vi "UI - Initiate Connection.vi"(8 "error in (no error)":errorcluster, 10 "Controller Address":string, 11 "Message Queue":refnum<queue>) -> (0 "error out":errorcluster, 1 "Connected?":bool, 3 "dup Message Queue":refnum<queue>)   [LabVIEW 2013]
uses:
  Message Queue/Message Cluster.ctl
  controls/Variable References.ctl
  Globals/Global - Configuration Options.vi
  Globals/Global - UI Stream and Variable Connections.vi
  Message Queue/Message Queue.lvlib
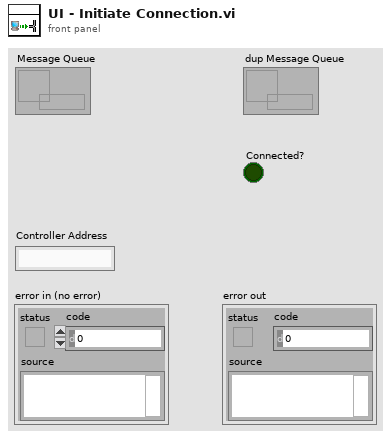
[diagram p1: front panel]
types:
  T1 = typedef "Message Queue.lvlib/Message Cluster.ctl" = cluster{"Message":string, "Message Data":variant}
  T2 = typedef "Variable References.ctl" = cluster{"CPU Usage":refnum<k21>, "Contiguous Memory":refnum<k21>, "Buffer Backlog":refnum<k21>, "Drive Space":refnum<k21>, "Number of Data Files":refnum<k21>, "System Time":refnum<k21>}
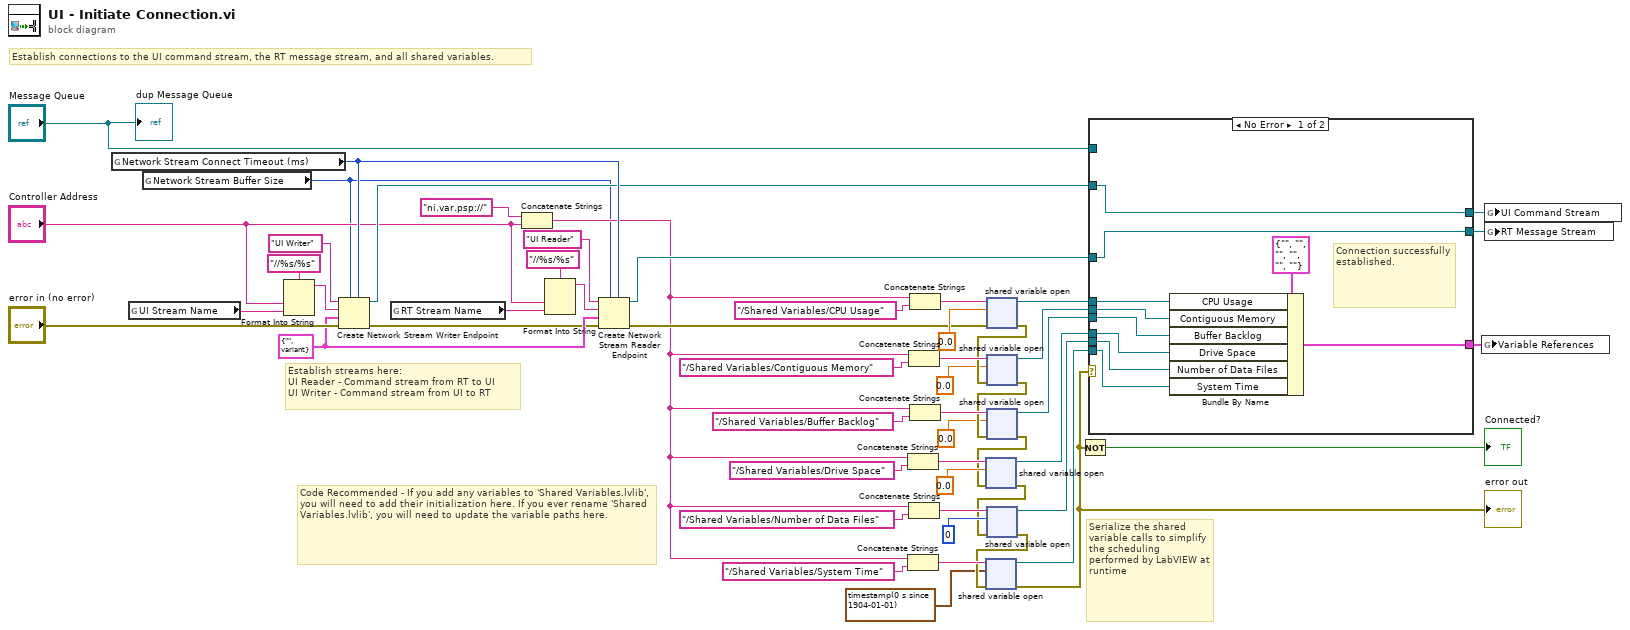
[diagram p0: block diagram]
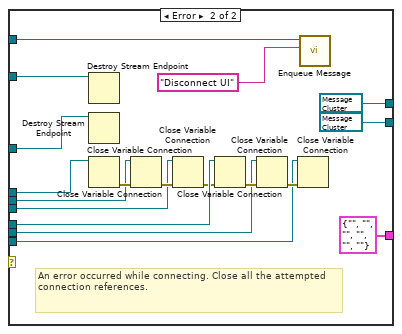
[diagram p2: hidden frame]
diagram:
  w44 = T1 {"Message"="", "Message Data"=variant} ("Message Cluster")
  # "Establish connections to the UI command stream, the RT message stream, and all shared variables."
  # "Code Recommended - If you add any variables to 'Shared Variables.lvlib', you will need to add their initialization here. If you ever rename 'Shared Variables.lvlib', you will need to update the variable paths here."
  # "Establish streams here:\nUI Reader - Command stream from RT to UI\nUI Writer - Command stream from UI to RT"
  # "Serialize the shared variable calls to simplify the scheduling performed by LabVIEW at runtime"
  n1 = global read "Global - Configuration Options.vi" "Network Stream Connect Timeout (ms)"() -> (w42:i32)
  n2 = global read "Global - Configuration Options.vi" "UI Stream Name"() -> (w49:string)
  n3 = global read "Global - Configuration Options.vi" "Network Stream Buffer Size"() -> (w3:i32)
  n4 = Format Into String(format string="//%s/%s", "Controller Address", w49) -> (resulting string=w48:string)  [unwired: 2 in, 1 out]
  n5 = Create Network Stream Writer Endpoint(5:w42, 7:w3, 8:"error in (no error)", 9:w44, 10:w48, 11:"UI Writer" ("reader name")) -> (0:w43:errorcluster, 3:w26:refnum<k21>)  [unwired: 1 in]
  n6 = global read "Global - Configuration Options.vi" "RT Stream Name"() -> (w52:string)
  n7 = Concatenate Strings("ni.var.psp://", "Controller Address") -> (w7:string)
  n8 = Format Into String(format string="//%s/%s", "Controller Address", w52) -> (resulting string=w51:string)  [unwired: 2 in, 1 out]
  n9 = Create Network Stream Reader Endpoint(5:w42, 7:w3, 8:w43, 9:w44, 10:w51, 11:"UI Reader" ("writer name")) -> (0:w39:errorcluster, 3:w27:refnum<k21>)  [unwired: 1 in]
  n10 = Concatenate Strings(w7, "/Shared Variables/Drive Space") -> (w19:string)
  n11 = Concatenate Strings(w7, "/Shared Variables/System Time") -> (w11:string)
  n12 = Concatenate Strings(w7, "/Shared Variables/Contiguous Memory") -> (w35:string)
  n13 = Concatenate Strings(w7, "/Shared Variables/Number of Data Files") -> (w14:string)
  n14 = Concatenate Strings(w7, "/Shared Variables/CPU Usage") -> (w38:string)
  n15 = Concatenate Strings(w7, "/Shared Variables/Buffer Backlog") -> (w34:string)
  n16 = shared-variable-open(w38, w39, 0.0) -> (w30:refnum<k21>, w32:errorcluster)  [unwired: 1 in]
  n17 = shared-variable-open(w35, w32, 0.0) -> (w29:refnum<k21>, w31:errorcluster)  [unwired: 1 in]
  n18 = shared-variable-open(w34, w31, 0.0) -> (w28:refnum<k21>, w2:errorcluster)  [unwired: 1 in]
  n19 = shared-variable-open(w19, w2, 0.0) -> (w18:refnum<k21>, w13:errorcluster)  [unwired: 1 in]
  n20 = shared-variable-open(w14, w13, u32 0) -> (w12:refnum<k21>, w10:errorcluster)  [unwired: 1 in]
  n21 = shared-variable-open(w11, w10, timestamp(0 s since 1904-01-01) ("time stamp")) -> (w8:refnum<k21>, w9:errorcluster)  [unwired: 1 in]
  "error out" <- w9
  n22 = Not(x=w9) -> (.not. x?=→"Connected?":bool)
  n23 = case shown="No Error" w9 {
    tunnel: w30 -> [w63 w78]
    tunnel: w29 -> [w62 w76]
    tunnel: w28 -> [w61 w77]
    tunnel: w27 -> [w58 w81]
    tunnel: w26 -> [w59 w82]
    tunnel: [w60 T2 {"CPU Usage"="", "Contiguous Memory"="", "Buffer Backlog"="", "Drive Space"="", "Number of Data Files"="", "System Time"=""} ("Variable References")] -> w25
    tunnel: [w59 refnum<k21> refnum] -> w24
    tunnel: [w58 refnum<k21> refnum] -> w23
    tunnel: w18 -> [w57 w74]
    tunnel: w12 -> [w56 w72]
    tunnel: w8 -> [w55 w70]
    tunnel: "Message Queue" -> [_ w67]
    frame No Error {
      # "Connection successfully established."
      n24 = Bundle By Name(cluster=T2 {"CPU Usage"="", "Contiguous Memory"="", "Buffer Backlog"="", "Drive Space"="", "Number of Data Files"="", "System Time"=""} ("Variable References"), "CPU Usage"=w63, "Contiguous Memory"=w62, "Buffer Backlog"=w61, "Drive Space"=w57, "Number of Data Files"=w56, "System Time"=w55) -> (w60:T2)
    }
    frame Error {
      # "An error occurred while connecting. Close all the attempted connection references."
      n25 = Destroy Stream Endpoint(11:w82) -> ()  [unwired: 1 in, 1 out]
      n26 = Destroy Stream Endpoint(11:w81) -> ()  [unwired: 1 in, 1 out]
      n27 = Close Variable Connection(11:w78) -> (0:w79:errorcluster)  [unwired: 1 in]
      n28 = Close Variable Connection(8:w79, 11:w76) -> (0:w80:errorcluster)
      n29 = Close Variable Connection(8:w80, 11:w77) -> (0:w65:errorcluster)
      n30 = Close Variable Connection(8:w65, 11:w74) -> (0:w73:errorcluster)
      n31 = Close Variable Connection(8:w73, 11:w72) -> (0:w71:errorcluster)
      n32 = Close Variable Connection(8:w71, 11:w70) -> ()  [unwired: 1 out]
      n33 = call "Enqueue Message.vi"("Message"="Disconnect UI", "Message Queue"=w67) -> ()  [unwired: 8 in, 2 out]
    }
  }
  n34 = global write "Global - UI Stream and Variable Connections.vi" "Variable References"(w25) -> ()
  n35 = global write "Global - UI Stream and Variable Connections.vi" "UI Command Stream"(w24) -> ()
  n36 = global write "Global - UI Stream and Variable Connections.vi" "RT Message Stream"(w23) -> ()
  "dup Message Queue" <- "Message Queue"
